vi "getRfCalibration.vi"(8 "error in (no error)":errorcluster, 11 "RfOutputChannel in":refnum<class "RfOutputChannel.lvclass">) -> (0 "error out":errorcluster, 2 "calibration":T1, 3 "RfOutputChannel out":refnum<class "RfOutputChannel.lvclass">)   [LabVIEW 2011, in "Tools.lvlib" / "DatabaseHelpers.lvlib" / "RfOutputChannel.lvclass"]
uses:
  RfOutputChannel.lvclass
  RfOutputChannel.lvclass/RfOutputChannel.ctl
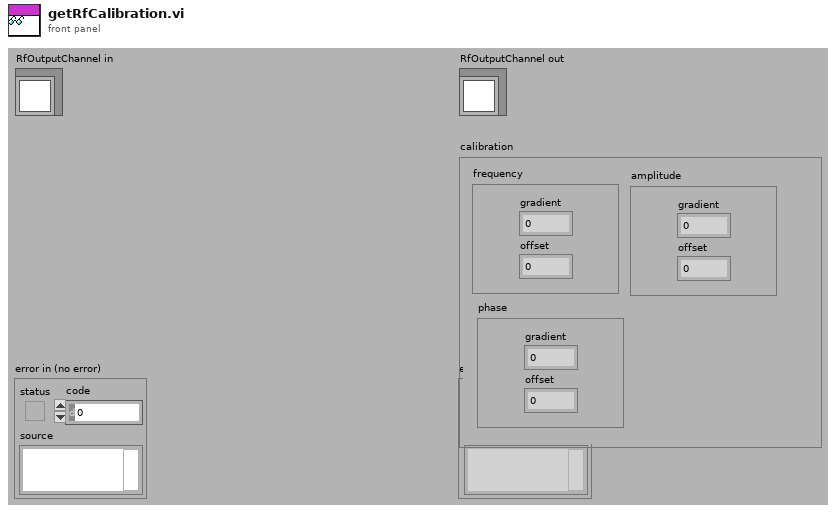
[diagram p1: front panel]
types:
  T1 = cluster{"frequency":cluster{"gradient":dbl, "offset":dbl}, "amplitude":cluster{"gradient":dbl, "offset":dbl}, "phase":cluster{"gradient":dbl, "offset":dbl}}
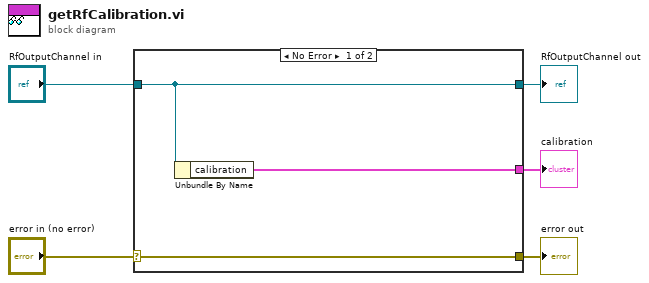
[diagram p0: block diagram]
diagram:
  n1 = case shown="No Error" "error in (no error)" {
    selector: "error in (no error)" -> [w8 w9]
    tunnel: [w8 w9] -> w4
    tunnel: [w7 w10] -> w2
    tunnel: "RfOutputChannel in" -> [w7 w10]
    tunnel: [w6 _] -> w1
    frame No Error {
      n2 = Unbundle By Name(w7) -> ("calibration"=w6:T1)
    }
    frame Error {
    }
  }
  "error out" <- w4
  "RfOutputChannel out" <- w2
  "calibration" <- w1
